vi "Find Contours.vi"(5 "Contour Approximation Mode (Default: SIMPLE)":T5=enum."SIMPLE", 7 "Contour Retrieval Modes (Default: TREE)":T4=enum."TREE", 8 "error in (no error)":errorcluster, 11 "Greyscale Image in":T6) -> (0 "error out":errorcluster, 2 "Found Contours":T1[](array[typedef]), 3 "Greyscale Image":T6)   [LabVIEW 2020, in "feature_detection.lvlib"]
doc: "Finds contours in a binary image. Detected contours can be further processed using functions such as Approximate Polygon.vi and Contour Conver Hull.vi."
uses:
  feature_detection.lvlib
  image/Greyscale Image.ctl
  Contour Approximation Mode.ctl
  Contour Retrieval Modes.ctl
  Found Contour.ctl
  common/Image Point (Integer).ctl
  Contour Hierarchy.ctl
  common/common.lvlib
  common/bin/gartoolkit_fd_32-1.dll
  image/image.lvlib
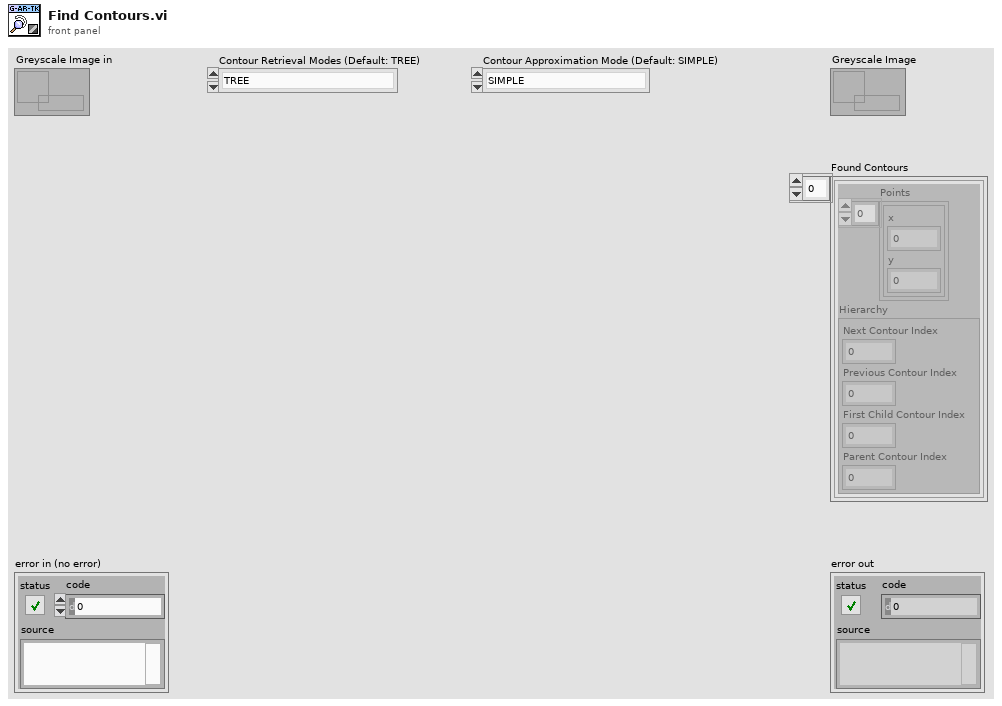
[diagram p1: front panel]
types:
  T1 = typedef "feature_detection.lvlib/Found Contour.ctl" = cluster{"Points":T2[], "Hierarchy":T3}
  T2 = typedef "common.lvlib/Image Point (Integer).ctl" = cluster{"x":i32, "y":i32}
  T3 = typedef "feature_detection.lvlib/Contour Hierarchy.ctl" = cluster{"Next Contour Index":i32, "Previous Contour Index":i32, "First Child Contour Index":i32, "Parent Contour Index":i32}
  T4 = typedef "feature_detection.lvlib/Contour Retrieval Modes.ctl" = enum16{"EXTERNAL", "LIST", "CCOMP", "TREE"}
  T5 = typedef "feature_detection.lvlib/Contour Approximation Mode.ctl" = enum16{"NONE", "SIMPLE", "TC89_L1", "TC89_KCOS"}
  T6 = typedef "image.lvlib/Greyscale Image.ctl" = refnum<data-value>
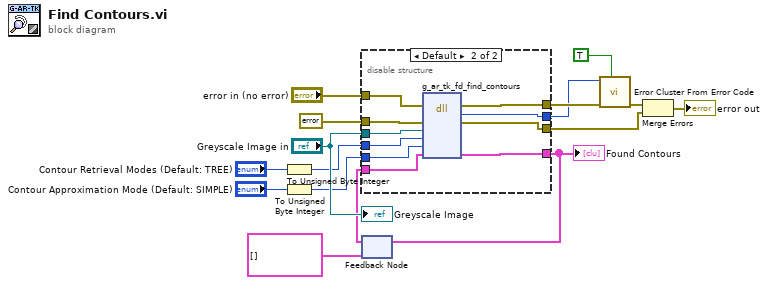
[diagram p0: block diagram]
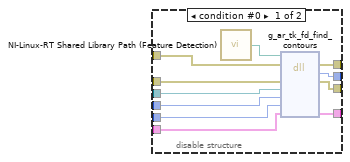
[diagram p2: hidden frame]
diagram:
  n1 = To Unsigned Byte Integer(number="Contour Retrieval Modes (Default: TREE)") -> (unsigned 8bit integer=w9:u8)
  n2 = To Unsigned Byte Integer(number="Contour Approximation Mode (Default: SIMPLE)") -> (unsigned 8bit integer=w8:u8)
  n3 = feedback #1(T1[] [] ("Array")) -> (w2:T1[])
  n4 = disable-structure shown="Default" {
    disable-tunnel: "error in (no error)" -> [w26 w37]
    disable-tunnel: errorcluster {"status"=FALSE, "code"=0, "source"=""} ("error constant") -> [w25 w36]
    disable-tunnel: "Greyscale Image in" -> [w24 w35]
    disable-tunnel: w9 -> [w23 w34]
    disable-tunnel: w8 -> [w22 w33]
    disable-tunnel: w2 -> [w21 w32]
    disable-tunnel: [w20 w31] -> w7
    disable-tunnel: [w19 w30] -> w6
    disable-tunnel: [w18 w29] -> w5
    disable-tunnel: [w17 w28] -> w3
    frame condition #0 {
      n5 = call "NI-Linux-RT Shared Library Path (Feature Detection).vi"() -> ("Path"=w27:path)
      n6 = dll-call lib="?" fn="g_ar_tk_fd_find_contours" ("g_ar_toolkit.*.*:g_ar_tk_image_draw_line")(path in=w27, error in=w26, "error_cluster"=w25, "EDVR src"=w24, "retrieval_mode"=w23, "contour_mode"=w22, "contours"=w21) -> (error out=w20:errorcluster, "mg_err_code"=w19:i32, "error_cluster"=w18:errorcluster, "contours"=w17:T1[])  [unwired: 4 in, 1 out]
    }
    frame condition #1 (active) {
      n7 = dll-call lib="C:/serenial/lib/g-augmented-reality-toolkit/LabVIEW/common/bin/gartoolkit_fd_*-1.*" fn="g_ar_tk_fd_find_contours" ("g_ar_toolkit.*.*:g_ar_tk_image_draw_line")(error in=w37, "error_cluster"=w36, "EDVR src"=w35, "retrieval_mode"=w34, "contour_mode"=w33, "contours"=w32) -> (error out=w31:errorcluster, "mg_err_code"=w30:i32, "error_cluster"=w29:errorcluster, "contours"=w28:T1[])  [unwired: 5 in, 1 out]
    }
  }
  "Found Contours" <- w3
  n8 = feedback-in #1(w3) -> ()
  n9 = call <vilib>:"Error Cluster From Error Code.vi"("show call chain? (False)"=TRUE, "error in (no error)"=w7, "error code (0)"=w6) -> ("error out"=w15:errorcluster)  [unwired: 6 in]
  n10 = Merge Errors(w15, w5) -> (→"error out":errorcluster)
  "Greyscale Image" <- "Greyscale Image in"
